vi "子VI-查看某框-不显示界面-只读穿透图模式.vi"(0 "框号":dbl format="%#_13g", 1 "框组":T3(array[cluster]), 2 "临界Z值":i32, 4 "临界面积百分比值":dbl, 5 "预先配置的灰度阈值":dbl, 6 "穿透图原始路径":path, 7 "部位信息":string[](array[string])=["", "34.500000", "32.500000", "1121", "34", "54.955926", "分层类", "不合格", ""], 12 "产品规格":cluster{"产品长度（周长）（mm）":dbl, "产品宽度（母线长）（mm）":dbl}) -> (14 "弥散类检测结果":string[][](table), 19 "分层类检测结果":string[][](table))   [LabVIEW 2018]
uses:
  <vilib>/vision/NI_Vision_Development_Module.lvlib
panel:
  in  "Tab Control":T1
  out "?":T2(plugin-control)
  out "Threshold Image":T2(plugin-control)
  out "Threshold Image":T2(plugin-control)
  in  "格式字符串 3":string="%f"
  in  "分隔符（'\\'代码显示） 2":string="\t"
  out "弥散和分层临界灰度值":i64
  out "弥散缺陷个数":i32
  out "分层缺陷个数":i32
  out "合格？ 弥散类":string="fencengThreshold"
  out "合格？分层类":string="fencengThreshold"
  out "弥散测量结果":dbl[][](array[numeric]) format="%.2f"
  out "面积 (pixels)":i32
  in  "格式字符串 2":string="%f"
  in  "分隔符（'\\'代码显示）":string="\t"
  out "分层测量结果":dbl[][](array[numeric]) format="%.2f"
  out "缺陷初步分类的临界值":sgl format="%#.3f"
  # "所选区域信息"
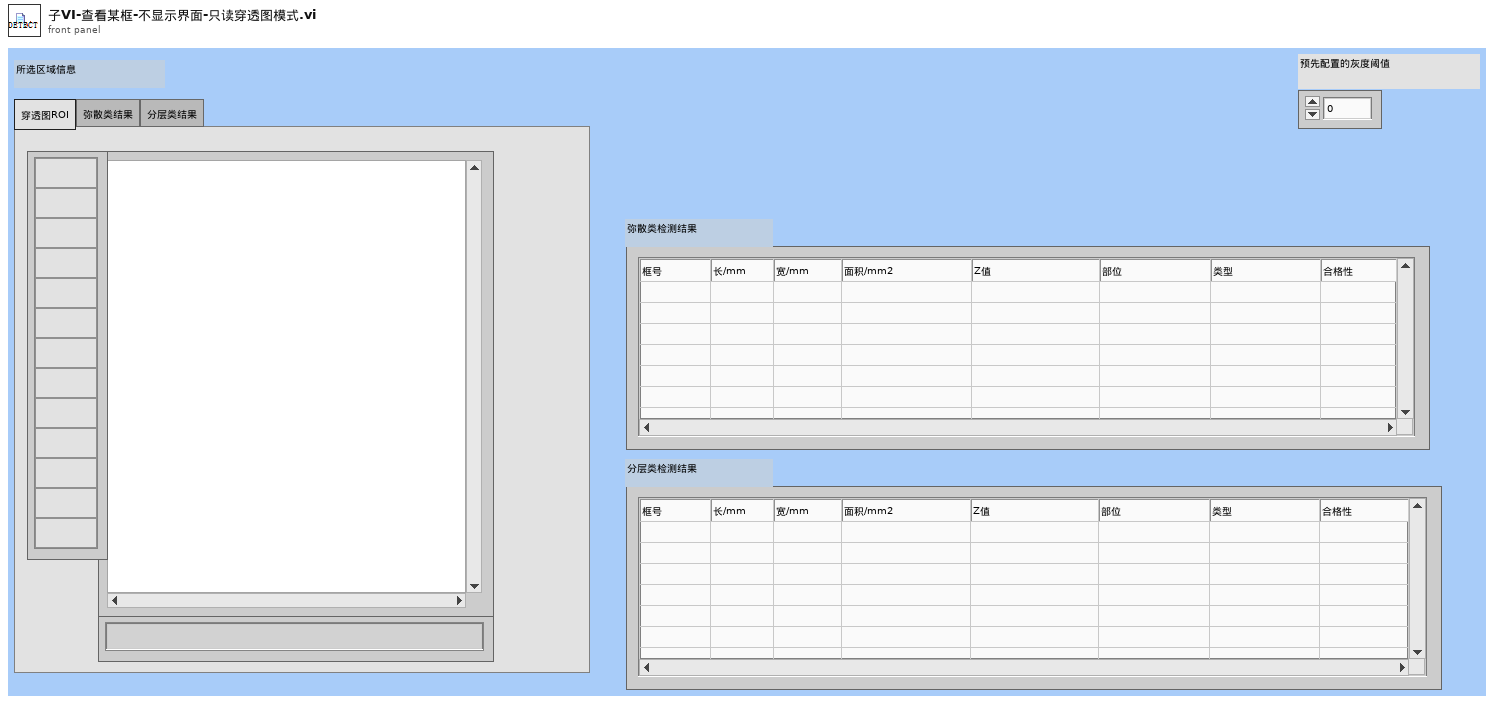
[diagram p1: front panel]
types:
  T1 = typedef "控件2.ctl" = enum32{"穿透图ROI", "弥散类结果", "分层类结果"}
  T2 = typedef "IMAQ Image.ctl" = refnum<image>
  T3 = cluster{"Global Rectangle":i32[], "Contours":cluster{"Contour Type":u32, "ROI Type":u32, "Points":i32[]}[]}[]
  T4 = typedef "Image Type" = u32
  T5 = typedef "Particle Parameters" = i32
  T6 = cluster{"Measurement Parameter":T5, "Range Lower Value":dbl, "Range Upper Value":dbl, "Range":bool, "Measurement Type":bool}[]
  T7 = cluster{"Global Rectangle":i32[], "Contours":cluster{"Contour Type":u32, "ROI Type":u32, "Points":i32[]}[]}
  T8 = cluster{"histogram":u32[], "Minimal Value":sgl, "Maximal Value":sgl, "Starting Value":sgl, "Interval Width":sgl, "Mean Value":sgl, "Standard  Variation":sgl, "Area (pixels)":i32}
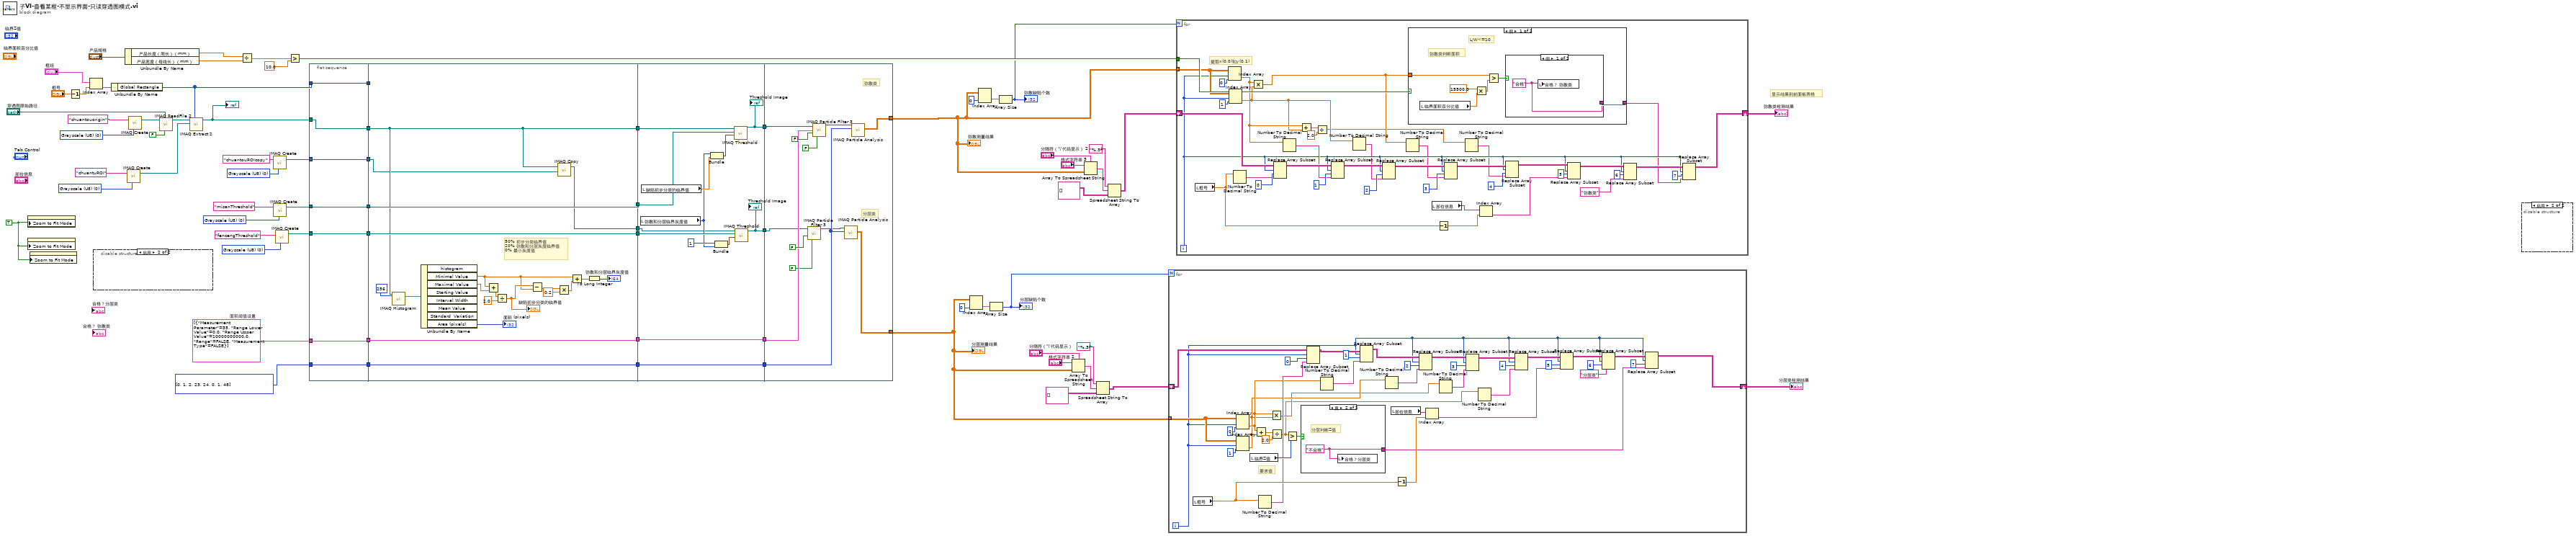
[diagram p0: block diagram]
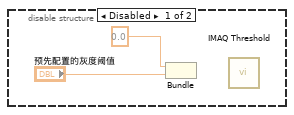
[diagram p2: hidden frame]
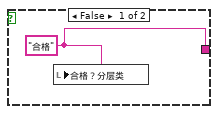
[diagram p3: hidden frame]
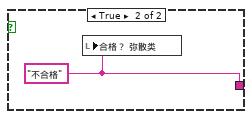
[diagram p4: hidden frame]
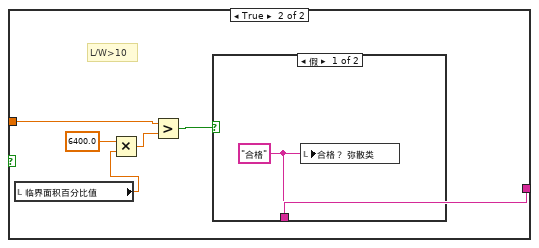
[diagram p5: hidden frame]
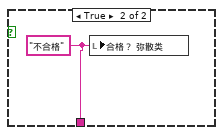
[diagram p6: hidden frame]
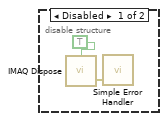
[diagram p7: hidden frame]
diagram:
  w1 = T4 0 items=["Grayscale (U8)", "Grayscale (I16)", "Grayscale (SGL)", "Complex (CSG)", "RGB (U32)", "HSL (U32)", "RGB (U64)", "Grayscale (U16)"] ("Image Type")
  w6 = TRUE ("Zoom to Fit Mode")
  w49 = T4 0 items=["Grayscale (U8)", "Grayscale (I16)", "Grayscale (SGL)", "Complex (CSG)", "RGB (U32)", "HSL (U32)", "RGB (U64)", "Grayscale (U16)"] ("Image Type")
  w50 = T4 0 items=["Grayscale (U8)", "Grayscale (I16)", "Grayscale (SGL)", "Complex (CSG)", "RGB (U32)", "HSL (U32)", "RGB (U64)", "Grayscale (U16)"] ("Image Type")
  w53 = T4 0 items=["Grayscale (U8)", "Grayscale (I16)", "Grayscale (SGL)", "Complex (CSG)", "RGB (U32)", "HSL (U32)", "RGB (U64)", "Grayscale (U16)"] ("Image Type")
  w29 = i32[] [0, 1, 2, 23, 24, 0, 1, 48] items=["Bounding Rect Width", "Bounding Rect Height"] ("Pixel Measurements")
  w33 = T6 [{"Measurement Parameter"=35, "Range Lower Value"=0.0, "Range Upper Value"=10000000000.0, "Range"=FALSE, "Measurement Type"=FALSE}]  # 面积阈值设置
  w67 = T4 0 items=["Grayscale (U8)", "Grayscale (I16)", "Grayscale (SGL)", "Complex (CSG)", "RGB (U32)", "HSL (U32)", "RGB (U64)", "Grayscale (U16)"] ("Image Type")
  # "显示结果到前面板表格"
  n1 = property class="ImageControl"("Zoom to Fit Mode"=w6) -> ()  [unwired: 2 in, 2 out]
  n2 = property class="ImageControl"("Zoom to Fit Mode"=w6) -> ()  [unwired: 2 in, 2 out]
  n3 = property class="ImageControl"("Zoom to Fit Mode"=w6) -> ()  [unwired: 2 in, 2 out]
  n4 = Decrement(x="框号") -> (x-1=w69:dbl)
  n5 = Index Array(array="框组", index=w69) -> (element=w70:T7)
  n6 = disable-structure shown="启用" {
    frame Disabled {
      n7 = Bundle(0.0, "预先配置的灰度阈值"="预先配置的灰度阈值") -> ()  [unwired: 1 in, 1 out]
      n8 = call "IMAQ Threshold"() -> ()  [unwired: 6 in, 6 out]
    }
    frame Enabled {
    }
  }
  n9 = Unbundle By Name(w70) -> ("Global Rectangle"=w44:i32[])
  n10 = Unbundle By Name("产品规格") -> ("产品长度（周长）（mm）"=w61:dbl, "产品宽度（母线长）（mm）"=w60:dbl)
  n11 = call "IMAQ Create"("Image Name"="chuantuROI", "Image Type"=w53) -> ("New Image"=w52:T2)  [unwired: 3 in, 1 out]
  n12 = call "IMAQ Create"("Image Name"="chuantouorigin", "Image Type"=w67) -> ("New Image"=w55:T2)  [unwired: 3 in, 1 out]
  n13 = call "IMAQ ReadFile 2"("Use File Path Image Type"=FALSE, "File Path"="穿透图原始路径", "Image"=w55) -> ("Image Out"=w56:T2)  [unwired: 4 in, 4 out]
  n14 = call "IMAQ Extract 2"("Optional Rectangle"=w44, "Image Dst"=w52, "Image Src"=w56) -> ("Image Dst Out"=w9:T2)  [unwired: 7 in, 1 out]
  "?" <- w9
  n15 = Divide(x=w61, y=w60) -> (x/y=w64:dbl)
  n16 = call "IMAQ Create"("Image Name"="chuantouROIcopy", "Image Type"=w1) -> ("New Image"=w4:T2)  [unwired: 3 in, 1 out]
  n17 = call "IMAQ Create"("Image Name"="misanThreshold", "Image Type"=w49) -> ("New Image"=w40:T2)  [unwired: 3 in, 1 out]
  n18 = call "IMAQ Create"("Image Name"="fencengThreshold", "Image Type"=w50) -> ("New Image"=w38:T2)  [unwired: 3 in, 1 out]
  n19 = Greater?(x=w64, y=10.0) -> (0:w59:bool)
  n20 = flat-sequence {
    tunnel: w44 -> [w81]
    tunnel: w9 -> [w76]
    tunnel: [w81] -> w43
    tunnel: w40 -> [w80]
    tunnel: [w80] -> w41
    tunnel: [w79] -> w39
    tunnel: w38 -> [w79]
    tunnel: [w78] -> w34
    tunnel: w33 -> [w78]
    tunnel: [w77] -> w30
    tunnel: w29 -> [w77]
    tunnel: [w76] -> w7
    tunnel: w4 -> [w75]
    tunnel: [w75] -> w3
    tunnel: [w101] -> w42
    tunnel: [w100] -> w37
    tunnel: [w95] -> w32
    tunnel: [w94] -> w28
    tunnel: w30 -> [w94]
    tunnel: w34 -> [w95]
    tunnel: w39 -> [w100]
    tunnel: w41 -> [w101]
    tunnel: w43 -> [_]
    tunnel: [w84] -> w8
    tunnel: w7 -> [w84]
    tunnel: [w83] -> w5
    tunnel: w3 -> [w82]
    tunnel: w42 -> [w114]
    tunnel: w37 -> [w113]
    tunnel: [w103] -> w36
    tunnel: [w104] -> w35
    tunnel: w32 -> [w112]
    tunnel: [w112] -> w31
    tunnel: w28 -> [w111]
    tunnel: [w111] -> w27
    tunnel: w8 -> [w105]
    tunnel: w5 -> [w102]
    tunnel: [w119] -> w12
    tunnel: [w124] -> w20
    tunnel: w36 -> [w115]
    tunnel: w35 -> [w116]
    tunnel: w31 -> [w123]
    tunnel: w27 -> [w122]
    frame #0 {
    }
    frame #1 {
      # "50% 初步分类临界值\n20% 弥散和分层灰度临界值\n0% 最小灰度值"
      n21 = call "IMAQ Histogram"("Number of Classes"=256, "Image"=w84) -> ("Histogram Report"=w98:T8)  [unwired: 8 in, 1 out]
      n22 = Unbundle By Name(w98) -> ("Minimal Value"=w86:sgl, "Maximal Value"=w92:sgl, "Area (pixels)"=→"面积 (pixels)":i32)  [unwired: 5 out]
      n23 = Add(x=w86, y=w92) -> (x+y=w91:sgl)
      n24 = Divide(x=w91, y=sgl 2.0) -> (x/y=w90:sgl)
      "缺陷初步分类的临界值" <- w90
      n25 = Subtract(x=w90, y=w86) -> (x-y=w88:sgl)
      n26 = Multiply(x=w88, y=0.2) -> (x*y=w87:dbl)
      n27 = call "IMAQ Copy"("Image Dst"=w82, "Image Src"=w84) -> ("Image Dst Out"=w83:T2)  [unwired: 4 in, 1 out]
      n28 = Add(x=w86, y=w87) -> (x+y=w85:dbl)
      n29 = To Long Integer(number=w85) -> (32bit integer=→"弥散和分层临界灰度值":i32)
    }
    frame #2 {
      n30 = local read "弥散和分层临界灰度值"() -> (w107:i64)
      n31 = local read "缺陷初步分类的临界值"() -> (w109:sgl)
      n32 = Bundle("弥散和分层临界灰度值"=w107, "缺陷初步分类的临界值"=w109) -> (w110:cluster{"弥散和分层临界灰度值":i64, "缺陷初步分类的临界值":sgl})  [unwired: 1 in]
      n33 = Bundle(1, "弥散和分层临界灰度值"=w107) -> (w106:cluster{i32, "弥散和分层临界灰度值":i64})  [unwired: 1 in]
      n34 = call "IMAQ Threshold"("Range"=w110, "Image Dst"=w114, "Image Src"=w105) -> ("Image Dst Out"=w104:T2)  [unwired: 3 in, 5 out]
      "Threshold Image" <- w104
      n35 = call "IMAQ Threshold"("Range"=w106, "Image Dst"=w113, "Image Src"=w102) -> ("Image Dst Out"=w103:T2)  [unwired: 3 in, 5 out]
      "Threshold Image" <- w103
    }
    frame #3 {
      # "分层类"
      # "弥散类"
      n36 = call "IMAQ Particle Filter 3"("Image Src"=w115, "Keep/Remove Particles (F)"=FALSE, "Reject Border? (F)"=FALSE) -> ("Image Dst Out"=w120:T2)  [unwired: 10 in, 2 out]
      n37 = call "IMAQ Particle Filter 3"("Image Src"=w116, "Selection Values"=w123, "Keep/Remove Particles (F)"=FALSE, "Reject Border? (F)"=FALSE) -> ("Image Dst Out"=w121:T2)  [unwired: 9 in, 2 out]
      n38 = call "IMAQ Particle Analysis"("Pixel Measurements"=w122, "Image"=w120) -> ("Particle Measurements (Pixels)"=w124:dbl[][])  [unwired: 4 in, 5 out]
      n39 = call "IMAQ Particle Analysis"("Pixel Measurements"=w122, "Image"=w121) -> ("Particle Measurements (Pixels)"=w119:dbl[][])  [unwired: 4 in, 5 out]
    }
  }
  n40 = Index Array(array=w20, index (col)=0 ("禁用的索引 (列)")) -> (element=w48:dbl[])  [unwired: 1 in]
  n41 = Index Array(array=w12, index (col)=0 ("禁用的索引 (列)")) -> (element=w46:dbl[])  [unwired: 1 in]
  n42 = Array Size(array=w48) -> (size(s)=w26:i32)
  "分层缺陷个数" <- w26
  n43 = Array Size(array=w46) -> (size(s)=w58:i32)
  "弥散缺陷个数" <- w58
  n44 = Array To Spreadsheet String(delimiter (Tab)="分隔符（'\\'代码显示）", array=w20, 3:"格式字符串 2") -> (spreadsheet string=w23:string)
  n45 = Array To Spreadsheet String(delimiter (Tab)="分隔符（'\\'代码显示） 2", array=w12, 3:"格式字符串 3") -> (spreadsheet string=w15:string)
  n46 = Spreadsheet String To Array(format string="%.3f", spreadsheet string=w23, array type (2D Dbl)=string[][] [] ("Array")) -> (array=w19:string[][])  [unwired: 1 in]
  n47 = Spreadsheet String To Array(format string="%.3f", spreadsheet string=w15, array type (2D Dbl)=string[][] [] ("Array")) -> (array=w11:string[][])  [unwired: 1 in]
  n48 = for {
    N: w26 -> [_]
    tunnel: w20 -> [w158]
    shift-right: [w136] -> w18
    shift-left: w19 -> [w147]
    i -> [w131]
    # "要求值"
    n49 = local read "框号"() -> (w156:dbl)
    n50 = Index Array(array=w158, index (row)=w131, index (col)=0 ("禁用的索引 (列)")) -> (element=w135:dbl)
    n51 = Index Array(array=w158, index (row)=w131, index (col)=1 ("禁用的索引 (列)")) -> (element=w134:dbl)
    n52 = local read "临界Z值"() -> (w164:i32)
    n53 = Add(x=w135, y=w134) -> (x+y=w165:dbl)
    n54 = Number To Decimal String(number=w156) -> (decimal integer string=w148:string)  [unwired: 1 in]
    n55 = Multiply(x=w135, y=w134) -> (x*y=w133:dbl)
    n56 = Divide(x=w165, y=2.0) -> (x/y=w130:dbl)
    n57 = Greater?(x=w130, y=w164) -> (0:w166:bool)
    n58 = case shown="真" w166 {
      tunnel: [w167 w168] -> w127
      frame False {
        w167 = "合格" ("合格？")
        n59 = local write "合格？分层类"(w167) -> ()
      }
      frame True {
        w168 = "不合格" ("合格？")
        # "分层判断Z值"
        n60 = local write "合格？分层类"(w168) -> ()
      }
    }
    n61 = Replace Array Subset(array=w147, new element=w148, index (row)=w131, index (col)=0 ("索引 (列)")) -> (w146:string[][])
    n62 = Number To Decimal String(number=w135) -> (decimal integer string=w145:string)  [unwired: 1 in]
    n63 = Replace Array Subset(array=w146, new element=w145, index (row)=w131, index (col)=1 ("索引 (列)")) -> (w143:string[][])
    n64 = Number To Decimal String(number=w134) -> (decimal integer string=w144:string)  [unwired: 1 in]
    n65 = local read "部位信息"() -> (w160:string[])
    n66 = Decrement(x=w156) -> (x-1=w159:dbl)
    n67 = Replace Array Subset(array=w143, new element=w144, index (row)=w131, index (col)=2 ("索引 (列)")) -> (w142:string[][])
    n68 = Index Array(array=w160, index=w159) -> (element=w129:string)
    n69 = Number To Decimal String(number=w133) -> (decimal integer string=w141:string)  [unwired: 1 in]
    n70 = Replace Array Subset(array=w142, new element=w141, index (row)=w131, index (col)=3 ("索引 (列)")) -> (w140:string[][])
    n71 = Number To Decimal String(number=w130) -> (decimal integer string=w132:string)  [unwired: 1 in]
    n72 = Replace Array Subset(array=w140, new element=w132, index (row)=w131, index (col)=4 ("索引 (列)")) -> (w139:string[][])
    n73 = Replace Array Subset(array=w139, new element=w129, index (row)=w131, index (col)=5 ("索引 (列)")) -> (w138:string[][])
    n74 = Replace Array Subset(array=w138, new element="分层类" ("新元素/子数组"), index (row)=w131, index (col)=6 ("索引 (列)")) -> (w137:string[][])
    n75 = Replace Array Subset(array=w137, new element=w127, index (row)=w131, index (col)=7 ("索引 (列)")) -> (w136:string[][])
  }
  "分层类检测结果" <- w18
  n76 = for {
    N: w58 -> [_]
    tunnel: w59 -> [w207]
    tunnel: w12 -> [w206]
    shift-right: [w186] -> w10
    shift-left: w11 -> [w194]
    i -> [w184]
    # "提取x(0,0)和y(0,1)"
    n77 = local read "框号"() -> (w172:dbl)
    n78 = Index Array(array=w206, index (row)=w184, index (col)=0 ("禁用的索引 (列)")) -> (element=w178:dbl)
    n79 = Index Array(array=w206, index (row)=w184, index (col)=1 ("禁用的索引 (列)")) -> (element=w177:dbl)
    n80 = Number To Decimal String(number=w172) -> (decimal integer string=w195:string)  [unwired: 1 in]
    n81 = Multiply(x=w178, y=w177) -> (x*y=w182:dbl)
    n82 = Replace Array Subset(array=w194, new element=w195, index (row)=w184, index (col)=0 ("索引 (列)")) -> (w193:string[][])
    n83 = Number To Decimal String(number=w178) -> (decimal integer string=w185:string)  [unwired: 1 in]
    n84 = Add(x=w178, y=w177) -> (x+y=w180:dbl)
    n85 = Divide(x=w180, y=2.0) -> (x/y=w176:dbl)
    n86 = Replace Array Subset(array=w193, new element=w185, index (row)=w184, index (col)=1 ("索引 (列)")) -> (w192:string[][])
    n87 = Number To Decimal String(number=w177) -> (decimal integer string=w183:string)  [unwired: 1 in]
    n88 = Replace Array Subset(array=w192, new element=w183, index (row)=w184, index (col)=2 ("索引 (列)")) -> (w191:string[][])
    n89 = Number To Decimal String(number=w182) -> (decimal integer string=w181:string)  [unwired: 1 in]
    n90 = case shown="假" w207 {
      tunnel: w182 -> [w213 w221]
      tunnel: [w211 w219] -> w169
      frame False {
        # "弥散类判断面积"
        # "L/W<=10"
        n91 = local read "临界面积百分比值"() -> (w209:dbl)
        n92 = Multiply(x=15500.0, y=w209) -> (x*y=w208:dbl)
        n93 = Greater?(x=w213, y=w208) -> (0:w212:bool)
        n94 = case shown="假" w212 {
          tunnel: [w214 w215] -> w211
          frame False {
            w214 = "合格" ("合格？")
            n95 = local write "合格？ 弥散类"(w214) -> ()
          }
          frame True {
            w215 = "不合格" ("合格？")
            n96 = local write "合格？ 弥散类"(w215) -> ()
          }
        }
      }
      frame True {
        # "L/W>10"
        n97 = local read "临界面积百分比值"() -> (w216:dbl)
        n98 = Multiply(x=6400.0, y=w216) -> (x*y=w218:dbl)
        n99 = Greater?(x=w221, y=w218) -> (0:w220:bool)
        n100 = case shown="假" w220 {
          tunnel: [w222 w223] -> w219
          frame False {
            w222 = "合格" ("合格？")
            n101 = local write "合格？ 弥散类"(w222) -> ()
          }
          frame True {
            w223 = "不合格" ("合格？")
            n102 = local write "合格？ 弥散类"(w223) -> ()
          }
        }
      }
    }
    n103 = local read "部位信息"() -> (w174:string[])
    n104 = Decrement(x=w172) -> (x-1=w173:dbl)
    n105 = Replace Array Subset(array=w191, new element=w181, index (row)=w184, index (col)=3 ("索引 (列)")) -> (w190:string[][])
    n106 = Number To Decimal String(number=w176) -> (decimal integer string=w175:string)  [unwired: 1 in]
    n107 = Index Array(array=w174, index=w173) -> (element=w171:string)
    n108 = Replace Array Subset(array=w190, new element=w175, index (row)=w184, index (col)=4 ("索引 (列)")) -> (w189:string[][])
    n109 = Replace Array Subset(array=w189, new element=w171, index (row)=w184, index (col)=5 ("索引 (列)")) -> (w188:string[][])
    n110 = Replace Array Subset(array=w188, new element="弥散类" ("新元素/子数组"), index (row)=w184, index (col)=6 ("索引 (列)")) -> (w187:string[][])
    n111 = Replace Array Subset(array=w187, new element=w169, index (row)=w184, index (col)=7 ("索引 (列)")) -> (w186:string[][])
  }
  "弥散类检测结果" <- w10
  n112 = disable-structure shown="启用" {
    frame Disabled {
      n113 = call "IMAQ Dispose"("All Images? (No)"=TRUE) -> ("error out"=w225:errorcluster)  [unwired: 5 in]
      n114 = call <vilib>:"Simple Error Handler.vi"("error in (no error)"=w225) -> ()  [unwired: 4 in, 5 out]
    }
    frame Enabled {
    }
  }
  "分层测量结果" <- w20
  "弥散测量结果" <- w12
